vi "Periodic Tasks.vi"(8 "error in":errorcluster) -> ()   [LabVIEW 2020]
doc: "This VI runs in parallel to other tasks. It can contain as many user-defined periodic loops as you need. These can carry out PID or other sorts of timed response."
uses:
  <vilib>/Rock Robotics/WPI/Utilities/WPI_GetSetVariantRefNum.vi
  <vilib>/Rock Robotics/WPI/ThirdParty/Phoenix-LabVIEW/CANCoder/Get/CTRE_Phoenix_CANcoder_GetSensorData.vi
panel:
  out "Absolute Position BL":dbl
  out "Absolute Position BR":dbl
  out "Absolute Position FL":dbl
  out "Absolute Position FR":dbl
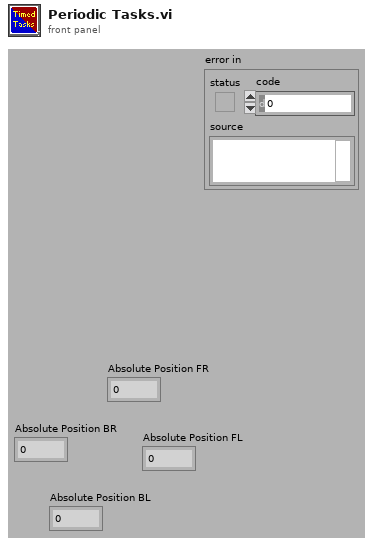
[diagram p1: front panel]
types:
  T1 = typedef "WPI_JoystickDevRef.ctl" = cluster{"Device":T2}
  T2 = typedef "WPI_JoystickDeviceEnum.ctl" = enum16{"USB 0", "USB 1", "USB 2", "USB 3", "USB 4", "USB 5"}
  T3 = typedef "CTRE_Phoenix_CANcoder_DeviceRef.ctl" = cluster{"DeviceStatus":errorcluster, "Device Number":u8, "Handle":u64, "UsageFrame":u32, "Library Path":path}
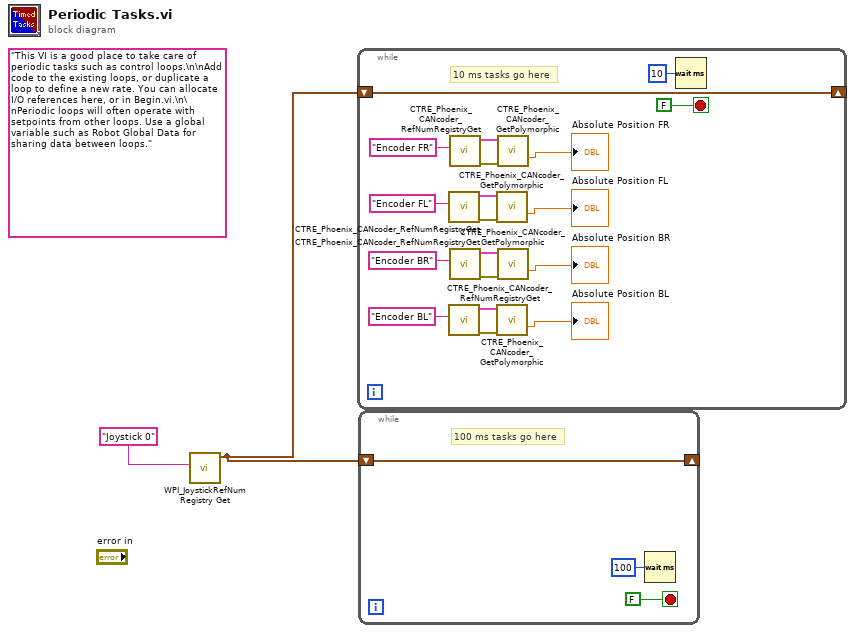
[diagram p0: block diagram]
diagram:
  (unwired) "This VI is a good place to take care of periodic tasks such as control loops.\n\nAdd code to the existing loops, or duplicate a loop to define a new rate. You can allocate I/O references here, or in Begin.vi.\n\nPeriodic loops will often operate with setpoints from other loops. Use a global variable such as Robot Global Data for sharing data between loops."
  n1 = call <vilib>:"WPI_JoystickRefNum Registry Get.vi"("refnum name"="Joystick 0") -> ("JoystickDevRef"=w1:T1)  [unwired: 1 in, 9 out]
  n2 = while {
    shift-right: [w19] -> _
    shift-left: w1 -> [w19]
    stop <- FALSE stop-if-true
    # "10 ms tasks go here"
    n3 = call <vilib>:"CTRE_Phoenix_CANcoder_RefNumRegistryGet.vi"("refnum name"="Encoder FL") -> ("error out"=w13:errorcluster, "CTRE_CANcoder_DeviceRef"=w14:T3)  [unwired: 9 in]
    n4 = call <vilib>:"CTRE_Phoenix_CANcoder_RefNumRegistryGet.vi"("refnum name"="Encoder BL") -> ("error out"=w5:errorcluster, "CTRE_CANcoder_DeviceRef"=w6:T3)  [unwired: 9 in]
    n5 = call <vilib>:"CTRE_Phoenix_CANcoder_RefNumRegistryGet.vi"("refnum name"="Encoder FR") -> ("error out"=w17:errorcluster, "CTRE_CANcoder_DeviceRef"=w18:T3)  [unwired: 9 in]
    n6 = call <vilib>:"CTRE_Phoenix_CANcoder_RefNumRegistryGet.vi"("refnum name"="Encoder BR") -> ("error out"=w9:errorcluster, "CTRE_CANcoder_DeviceRef"=w10:T3)  [unwired: 9 in]
    n7 = call-poly <vilib>:"CTRE_Phoenix_CANcoder_GetPolymorphic.vi"("CTRE_CANcoder_DeviceRef"=w14, "error in"=w13) -> ("Absolute Position"=→"Absolute Position FL":dbl)  [unwired: 9 in, 4 out]
    n8 = call-poly <vilib>:"CTRE_Phoenix_CANcoder_GetPolymorphic.vi"("CTRE_CANcoder_DeviceRef"=w6, "error in"=w5) -> ("Absolute Position"=→"Absolute Position BL":dbl)  [unwired: 9 in, 4 out]
    n9 = call-poly <vilib>:"CTRE_Phoenix_CANcoder_GetPolymorphic.vi"("CTRE_CANcoder_DeviceRef"=w18, "error in"=w17) -> ("Absolute Position"=→"Absolute Position FR":dbl)  [unwired: 9 in, 4 out]
    n10 = call-poly <vilib>:"CTRE_Phoenix_CANcoder_GetPolymorphic.vi"("CTRE_CANcoder_DeviceRef"=w10, "error in"=w9) -> ("Absolute Position"=→"Absolute Position BR":dbl)  [unwired: 9 in, 4 out]
    n11 = Wait (ms)(milliseconds to wait=u32 10) -> ()  [unwired: 1 out]
  }
  n12 = while {
    shift-right: [w22] -> _
    shift-left: w1 -> [w22]
    stop <- FALSE stop-if-true
    # "100 ms tasks go here"
    n13 = Wait (ms)(milliseconds to wait=u32 100) -> ()  [unwired: 1 out]
  }
